vi "VWFilpperPoly.vi"   [LabVIEW 2013]
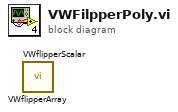
[diagram p0: block diagram]
diagram:
  n1 = call "VWflipperScalar.vi"() -> ()  [unwired: 11 in, 1 out]
  n2 = call "VWflipperArray.vi"() -> ()  [unwired: 11 in, 1 out]
